vi "Memory.Array.Bounds Check.Index.vi"(8 "error in (no error)":errorcluster, 10 "index":u64, 11 "Array in":refnum<class "Memory.Array.lvclass">) -> (0 "error out":errorcluster, 1 "index valid":bool, 2 "index out":u64, 3 "Array out":refnum<class "Memory.Array.lvclass">)   [LabVIEW 2016, in "LabVIEW Memory Manager.lvlib" / "Memory.Array.lvclass"]
uses:
  Memory.Array.lvclass
  Memory.Array.lvclass/Memory.Array.ctl
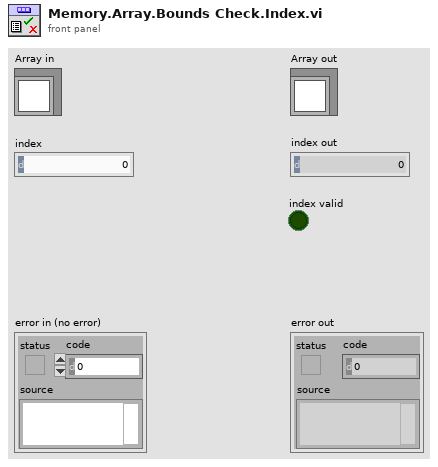
[diagram p1: front panel]
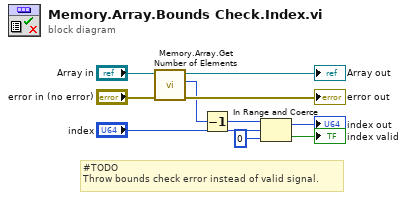
[diagram p0: block diagram]
diagram:
  # "#TODO\nThrow bounds check error instead of valid signal."
  n1 = call "Memory.Array.Get Number of Elements.vi"("error in (no error)"="error in (no error)", "Memory.Array in"="Array in") -> ("error out"=→"error out":errorcluster, "number of elements"=w2:u64, "Memory.Array out"=→"Array out":refnum<class "Memory.Array.lvclass">)  [unwired: 7 in]
  n2 = Decrement(x=w2) -> (x-1=w9:u64)
  n3 = In Range and Coerce(upper limit=w9, x="index", lower limit=u64 0) -> (coerced(x)=→"index out":u64, In Range?=→"index valid":bool)
